vi "Display External Document.vi"(8 "error in (no error)":errorcluster, 11 "Document Path":path) -> (0 "error out":errorcluster)   [LabVIEW 2013]
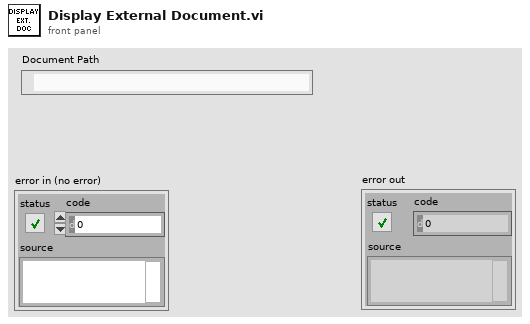
[diagram p1: front panel]
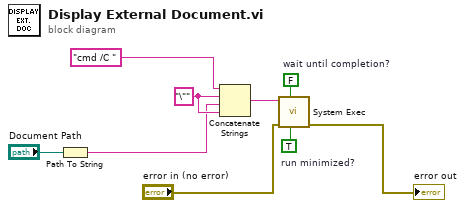
[diagram p0: block diagram]
diagram:
  w3 = TRUE  # run minimized?
  w4 = FALSE  # wait until completion?
  w8 = "\"" ("string")
  n1 = Path To String(path="Document Path") -> (string=w6:string)
  n2 = Concatenate Strings("cmd /C " ("command line"), w8, w6, w8) -> (w5:string)
  n3 = call <vilib>:"System Exec.vi"("run minimized? (F)"=w3, "wait until completion? (T)"=w4, "error in (no error)"="error in (no error)", "command line"=w5) -> ("error out"=→"error out":errorcluster)  [unwired: 2 in, 5 out]
